vi "Exercise 3-6.vi"() -> ()   [LabVIEW 2014]
panel:
  in  "End Conversions":bool
  in  "Type of Conversion":T1(ring)
  out "Output Temperature":dbl
  in  "Input Temperature":dbl
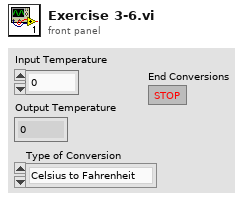
[diagram p1: front panel]
types:
  T1 = enum16{"Celsius to Fahrenheit", "Fahrenheit to Celsius", "Celsius to Kelvin", "Fahrenheit to Kelvin"}
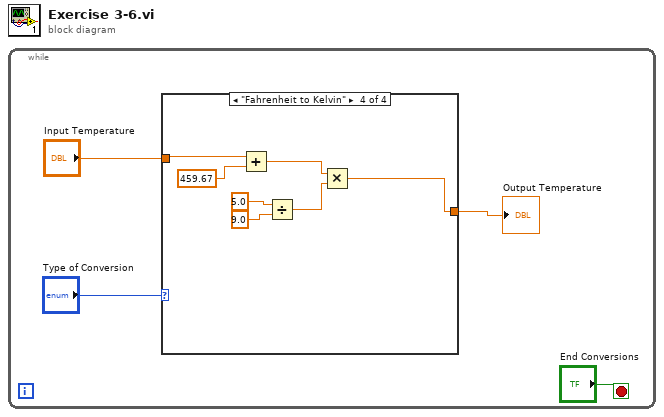
[diagram p0: block diagram]
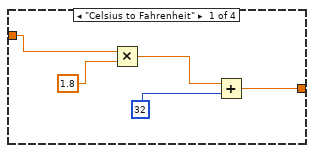
[diagram p2: hidden frame]
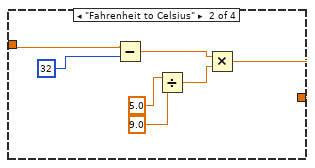
[diagram p3: hidden frame]
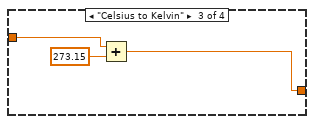
[diagram p4: hidden frame]
diagram:
  n1 = while {
    stop <- "End Conversions" stop-if-true
    n2 = case shown="\"Fahrenheit to Kelvin\"" "Type of Conversion" {
      tunnel: "Input Temperature" -> [w9 w16 w19 w26]
      tunnel: [w5 w10 w17 w22] -> w2
      frame "Celsius to Fahrenheit" {
        n3 = Multiply(x=w9, y=1.8) -> (x*y=w7:dbl)
        n4 = Add(x=w7, y=32) -> (x+y=w5:dbl)
      }
      frame "Fahrenheit to Celsius" {
        n5 = Subtract(x=w16, y=32) -> (x-y=w14:dbl)
        n6 = Divide(x=5.0, y=9.0) -> (x/y=w11:dbl)
        n7 = Multiply(x=w14, y=w11) -> (x*y=w10:dbl)
      }
      frame "Celsius to Kelvin" {
        n8 = Add(x=w19, y=273.15) -> (x+y=w17:dbl)
      }
      frame "Fahrenheit to Kelvin" {
        n9 = Add(x=w26, y=459.67) -> (x+y=w23:dbl)
        n10 = Divide(x=5.0, y=9.0) -> (x/y=w24:dbl)
        n11 = Multiply(x=w23, y=w24) -> (x*y=w22:dbl)
      }
    }
    "Output Temperature" <- w2
  }
